vi "TextToArrayTest.vi"(11 "error in":errorcluster) -> (15 "error out":errorcluster)   [LabVIEW 2023, in "TestVIs.lvlib"]
uses:
  TestVIs.lvlib
  <vilib>/addons/_JKI Toolkits/Caraya/classes/Assert/Assert Equal Value_Variant.vi
  <vilib>/addons/_JKI Toolkits/Caraya/classes/Test/Test.lvclass
  <vilib>/addons/_JKI Toolkits/Caraya/classes/Assert/Assert.lvclass
  Library/Unit Testing CA1.lvlib
panel:
  # "TEXT TO ARRAY TEST"
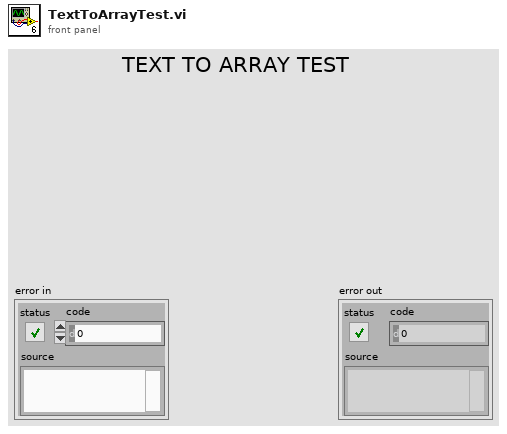
[diagram p1: front panel]
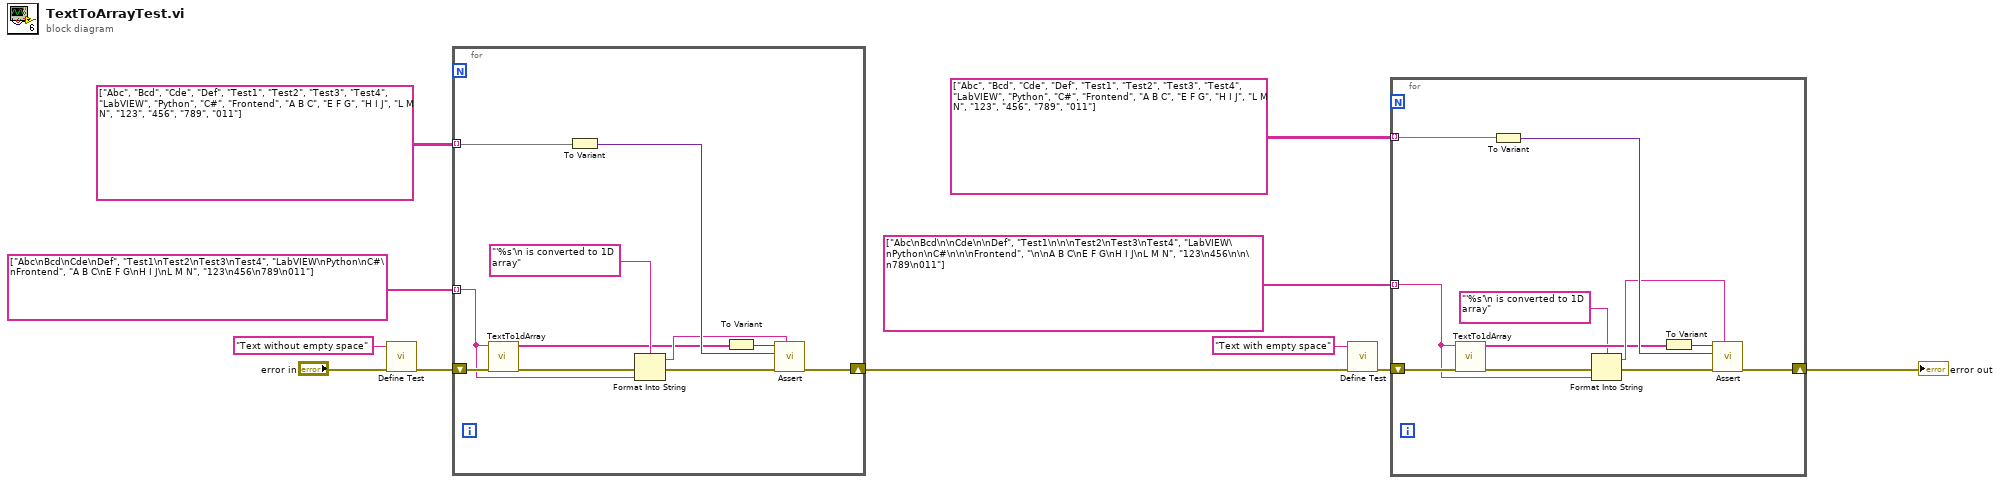
[diagram p0: block diagram]
diagram:
  n1 = call <vilib>:"Define Test.vi"("error in (no error)"="error in", "Label (VI Title)"="Text without empty space") -> ("error out"=w9:errorcluster)  [unwired: 8 in, 1 out]
  n2 = for {
    shift-right: [w16] -> w4
    shift-left: w9 -> [w15]
    tunnel: string[] ["Abc\nBcd\nCde\nDef", "Test1\nTest2\nTest3\nTest4", "LabVIEW\nPython\nC#\nFrontend", "A B C\nE F G\nH I J\nL M N", "123\n456\n789\n011"] ("Input Array") -> [w12] mode=indexing
    tunnel: string[][] [["Abc", "Bcd", "Cde", "Def"], ["Test1", "Test2", "Test3", "Test4"], ["LabVIEW", "Python", "C#", "Frontend"], ["A B C", "E F G", "H I J", "L M N"], ["123", "456", "789", "011"]] ("Input Array") -> [w17] mode=indexing
    n3 = call "TextTo1dArray.vi"("input string"=w12, "error in"=w15) -> ("Array"=w13:string[], "error out"=w14:errorcluster)  [unwired: 12 in]
    n4 = To Variant(anything=w17) -> (Variant=w22:variant)
    n5 = Format Into String(format string="'%s'\n is converted to 1D array", error in=w14, w12) -> (resulting string=w18:string, error out=w20:errorcluster)  [unwired: 1 in]
    n6 = To Variant(anything=w13) -> (Variant=w21:variant)
    n7 = call-poly <vilib>:"Assert.vi"("Label"=w18, "error in (no error)"=w20, "Y"=w22, "X"=w21) -> ("error out"=w16:errorcluster)  [unwired: 6 in, 1 out]
  }
  n8 = call <vilib>:"Define Test.vi"("error in (no error)"=w4, "Label (VI Title)"="Text with empty space") -> ("error out"=w5:errorcluster)  [unwired: 8 in, 1 out]
  n9 = for {
    shift-right: [w29] -> w3
    shift-left: w5 -> [w28]
    tunnel: string[] ["Abc\nBcd\n\nCde\n\nDef", "Test1\n\n\nTest2\nTest3\nTest4", "LabVIEW\nPython\nC#\n\n\nFrontend", "\n\nA B C\nE F G\nH I J\nL M N", "123\n456\n\n\n789\n011"] ("Input Array") -> [w23] mode=indexing
    tunnel: string[][] [["Abc", "Bcd", "Cde", "Def"], ["Test1", "Test2", "Test3", "Test4"], ["LabVIEW", "Python", "C#", "Frontend"], ["A B C", "E F G", "H I J", "L M N"], ["123", "456", "789", "011"]] ("Input Array") -> [w25] mode=indexing
    n10 = call "TextTo1dArray.vi"("input string"=w23, "error in"=w28) -> ("Array"=w26:string[], "error out"=w27:errorcluster)  [unwired: 12 in]
    n11 = To Variant(anything=w25) -> (Variant=w33:variant)
    n12 = Format Into String(format string="'%s'\n is converted to 1D array", error in=w27, w23) -> (resulting string=w30:string, error out=w31:errorcluster)  [unwired: 1 in]
    n13 = To Variant(anything=w26) -> (Variant=w32:variant)
    n14 = call-poly <vilib>:"Assert.vi"("Label"=w30, "error in (no error)"=w31, "Y"=w33, "X"=w32) -> ("error out"=w29:errorcluster)  [unwired: 6 in, 1 out]
  }
  "error out" <- w3
